vi "Test_interface.vi"() -> ()   [LabVIEW 2016]
uses:
  <vilib>/httpClient/POSTBuffer.vi
  <vilib>/httpClient/LabVIEWHTTPClient.lvlib
panel:
  in  "Address":string="10.0.1.201"
  out "value out":T1
  in  "url":string="hello"
  out "value in":T1
  out "JSON string":string
  out "length":i32
  out "headers":string
  out "body":string
  out "error out":errorcluster
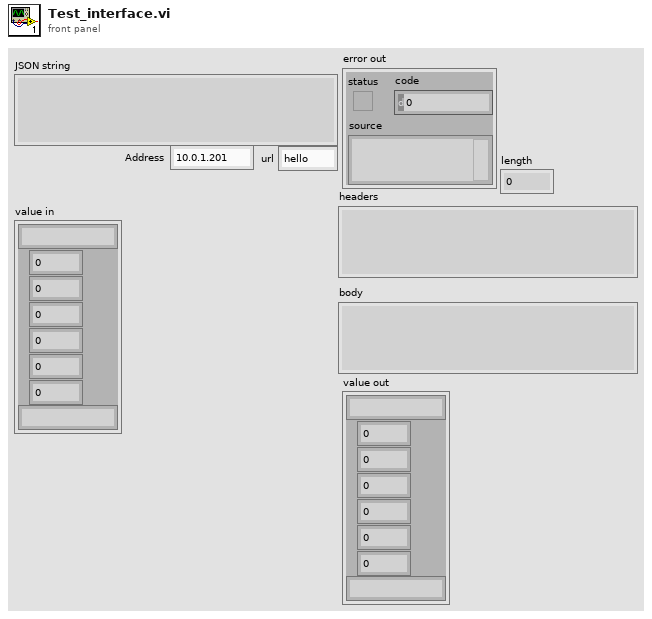
[diagram p1: front panel]
types:
  T1 = cluster{string, dbl, dbl, dbl, dbl, dbl, dbl, string}
  T2 = cluster{"name":string, "d1":dbl, "d2":dbl, "d3":dbl, "d4":dbl, "d5":dbl, "d6":dbl, "endstr":string}
  T3 = typedef "LabVIEWHTTPClient.lvlib/ClientHandle.ctl" = refnum<k1>
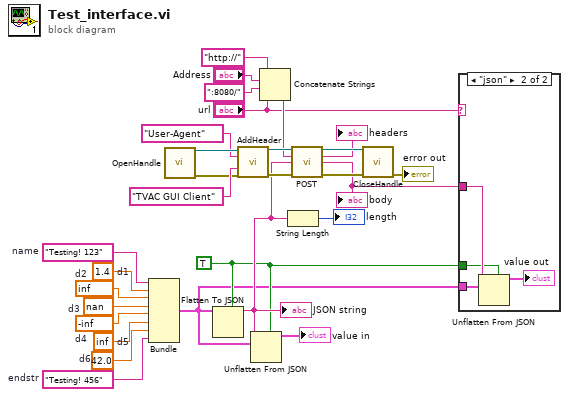
[diagram p0: block diagram]
diagram:
  w22 = "Testing! 456"  # endstr
  w5 = TRUE ("enable LabVIEW extensions? (T)")
  w23 = 42.0  # d6
  w24 = inf  # d5
  w26 = nan  # d3
  w25 = -inf  # d4
  w29 = "Testing! 123"  # name
  w28 = 1.4  # d1
  w27 = inf  # d2
  n1 = Bundle("name"=w29, "d1"=w28, "d2"=w27, "d3"=w26, "d4"=w25, "d5"=w24, "d6"=w23, "endstr"=w22) -> (w4:T2)  [unwired: 1 in]
  n2 = call <vilib>:"OpenHandle.vi"() -> ("client handle out"=w21:T3, "error out"=w18:errorcluster)  [unwired: 14 in]
  n3 = Flatten To JSON(enable LabVIEW extensions? (T)=w5, anything=w4) -> (JSON string=w8:string)  [unwired: 1 in, 1 out]
  "JSON string" <- w8
  n4 = call <vilib>:"AddHeader.vi"("client handle"=w21, "header"="User-Agent", "value"="TVAC GUI Client", "error in (no error)"=w18) -> ("client handle out"=w16:T3, "error out"=w17:errorcluster)  [unwired: 10 in]
  n5 = Unflatten From JSON(enable LabVIEW extensions? (T)=w5, JSON string=w8, type and defaults=w4) -> (value=→"value in":T2)  [unwired: 4 in, 1 out]
  n6 = Concatenate Strings("http://" ("url"), "Address", ":8080/" ("url"), "url") -> (w7:string)
  n7 = String Length(string=w8) -> (length=→"length":i32)
  n8 = call-poly <vilib>:"POST.vi"("client handle"=w16, "url"=w7, "buffer"=w8, "error in (no error)"=w17) -> ("client handle out"=w14:T3, "headers"=→"headers":string, "body"=w6:string, "error out"=w13:errorcluster)  [unwired: 8 in]
  "body" <- w6
  n9 = call <vilib>:"CloseHandle.vi"("client handle"=w14, "error in (no error)"=w13) -> ("error out"=→"error out":errorcluster)  [unwired: 13 in]
  n10 = case shown="\"json\"" "url" {
    tunnel: w6 -> [_ w33]
    tunnel: w5 -> [_ w32]
    tunnel: w4 -> [_ w31]
    frame "False", Default {
    }
    frame "json" {
      n11 = Unflatten From JSON(enable LabVIEW extensions? (T)=w32, JSON string=w33, type and defaults=w31) -> (value=→"value out":T2)  [unwired: 4 in, 1 out]
    }
  }
